vi "cycle_step_indicator.vi"() -> ()   [LabVIEW 2015]
panel:
  in  "Numeric":dbl
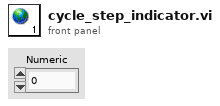
[diagram p1: front panel]
diagram:
